vi "read_and_write.vi"() -> ()   [LabVIEW 2017]
uses:
  <vilib>/Platform/TimedLoop/XDataNode/timing_clust.ctl
  <vilib>/Platform/TimedLoop/XDataNode/nitl_modes.ctl
  <vilib>/Platform/TimedLoop/XDataNode/wakeup.ctl
  <vilib>/rvi/Emulation/niFpgaSctlEmulationGetInTimedLoop.vi
  <vilib>/rvi/Emulation/niFpgaProcessEmulError.vi
  <vilib>/rvi/Emulation/niFpgaGetClockAttributes.vi
  <vilib>/rvi/Emulation/niFpgaEmulationReportErrorSimple.vi
  <vilib>/rvi/eio/common/nirviEmuTemplateMethod_errors.vi
  <vilib>/rvi/interface/RandomDataEmulation/niFpgaRandomDataHandleErrors.vi
  <vilib>/rvi/Emulation/niFpgaCriticalErrorInLSC.vi
  <vilib>/eio/EIONode/EIONode.xnode
  <vilib>/rvi/DataTransferAndStorage/Container/XNode/niFpgaContainer.xnode
  <vilib>/rvi/interface/RandomDataEmulation/nirviRandomDataFpgaReadWriteTemplate.vi
  <vilib>/Platform/TimedLoop/XDataNode/XDataNode.xnode
  <vilib>/Platform/TimedLoop/XDataNode/XDNodeRunTimeDep.lvlib
panel:
  in  "stop":bool
  in  "safety catch":bool=TRUE
  in  "Timeout scope":i32
  out "timed out scope":bool=TRUE
  in  "power threshold (scope)":i32=80
  out "trigger":i16
  in  "count ticks scope":u32=8500
  in  "count ticks generating":u32=50000
  in  "Timeout err_check":i32
  in  "Timeout gen":i32
  out "timed out error_check":bool
  in  "count ticks reading":u32=500
  in  "minus x channel (gen)":i16
  in  "minus y channel (gen)":i16
  out "timed out gen":bool=TRUE
  in  "power (gen)":i16
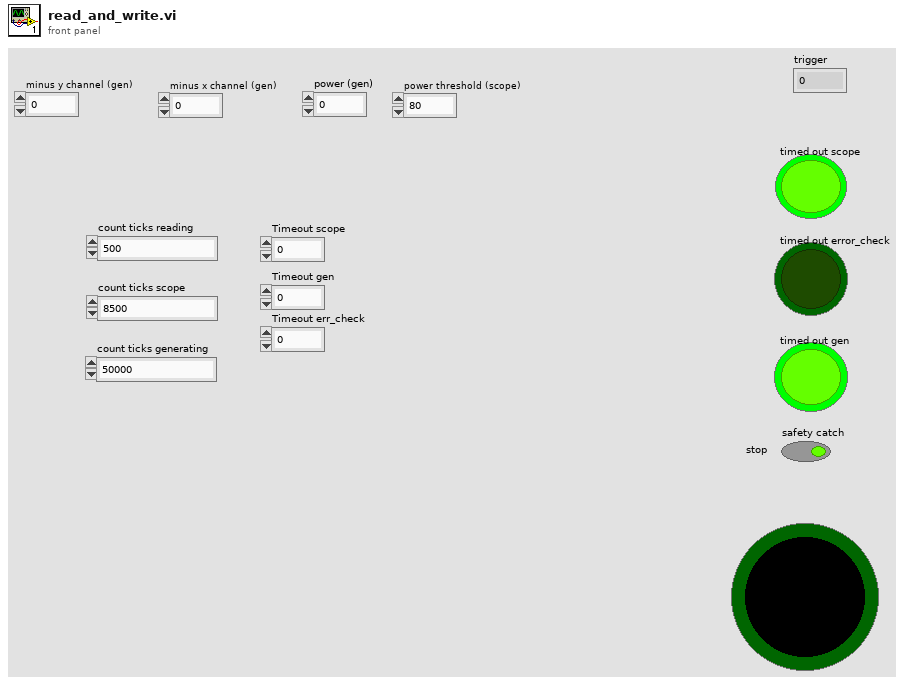
[diagram p1: front panel]
types:
  T1 = typedef "XDNodeRunTimeDep.lvlib/timing_clust.ctl" = cluster{"Expected End [f-1]":u64, "Actual End [f-1]":u64, "Finished Late? [f-1]":bool, "Expected End [i-1]":u64, "Actual End [i-1]":u64, "Finished Late? [i-1]":bool, "Expected Start [i]":u64, "Actual Start [i]":u64, "Expected Start [f]":u64, "Actual Start [f]":u64, "Source Name":string, "Structure Name":string, "Period":i64, "Deadline":i64, "Offset":i64, "Start":i64, "Priority":i32, "Timeout":i32, "Mode":T2, "Wakeup Reason":T3, "Error":errorcluster, "Source Type":string, "Secondary Source Type":string, "Global End Time":u64, "Global Start Time":u64, "Frame Duration":u64, "Iteration Duration":u64, "Assigned CPU":i32, "I/O Scan Engine Mode":u32}
  T2 = typedef "XDNodeRunTimeDep.lvlib/nitl_modes.ctl" = enum32{"No Change", "Process missed periods, maintain original phase", "Discard missed periods, maintain original phase", "Process missed periods, ignore original phase", "Discard missed periods, ignore original phase"}
  T3 = typedef "XDNodeRunTimeDep.lvlib/wakeup.ctl" = enum32{"Normal", "Aborted", "Asynchronous wakeup", "Timing source error", "Timed loop error", "Timeout"}
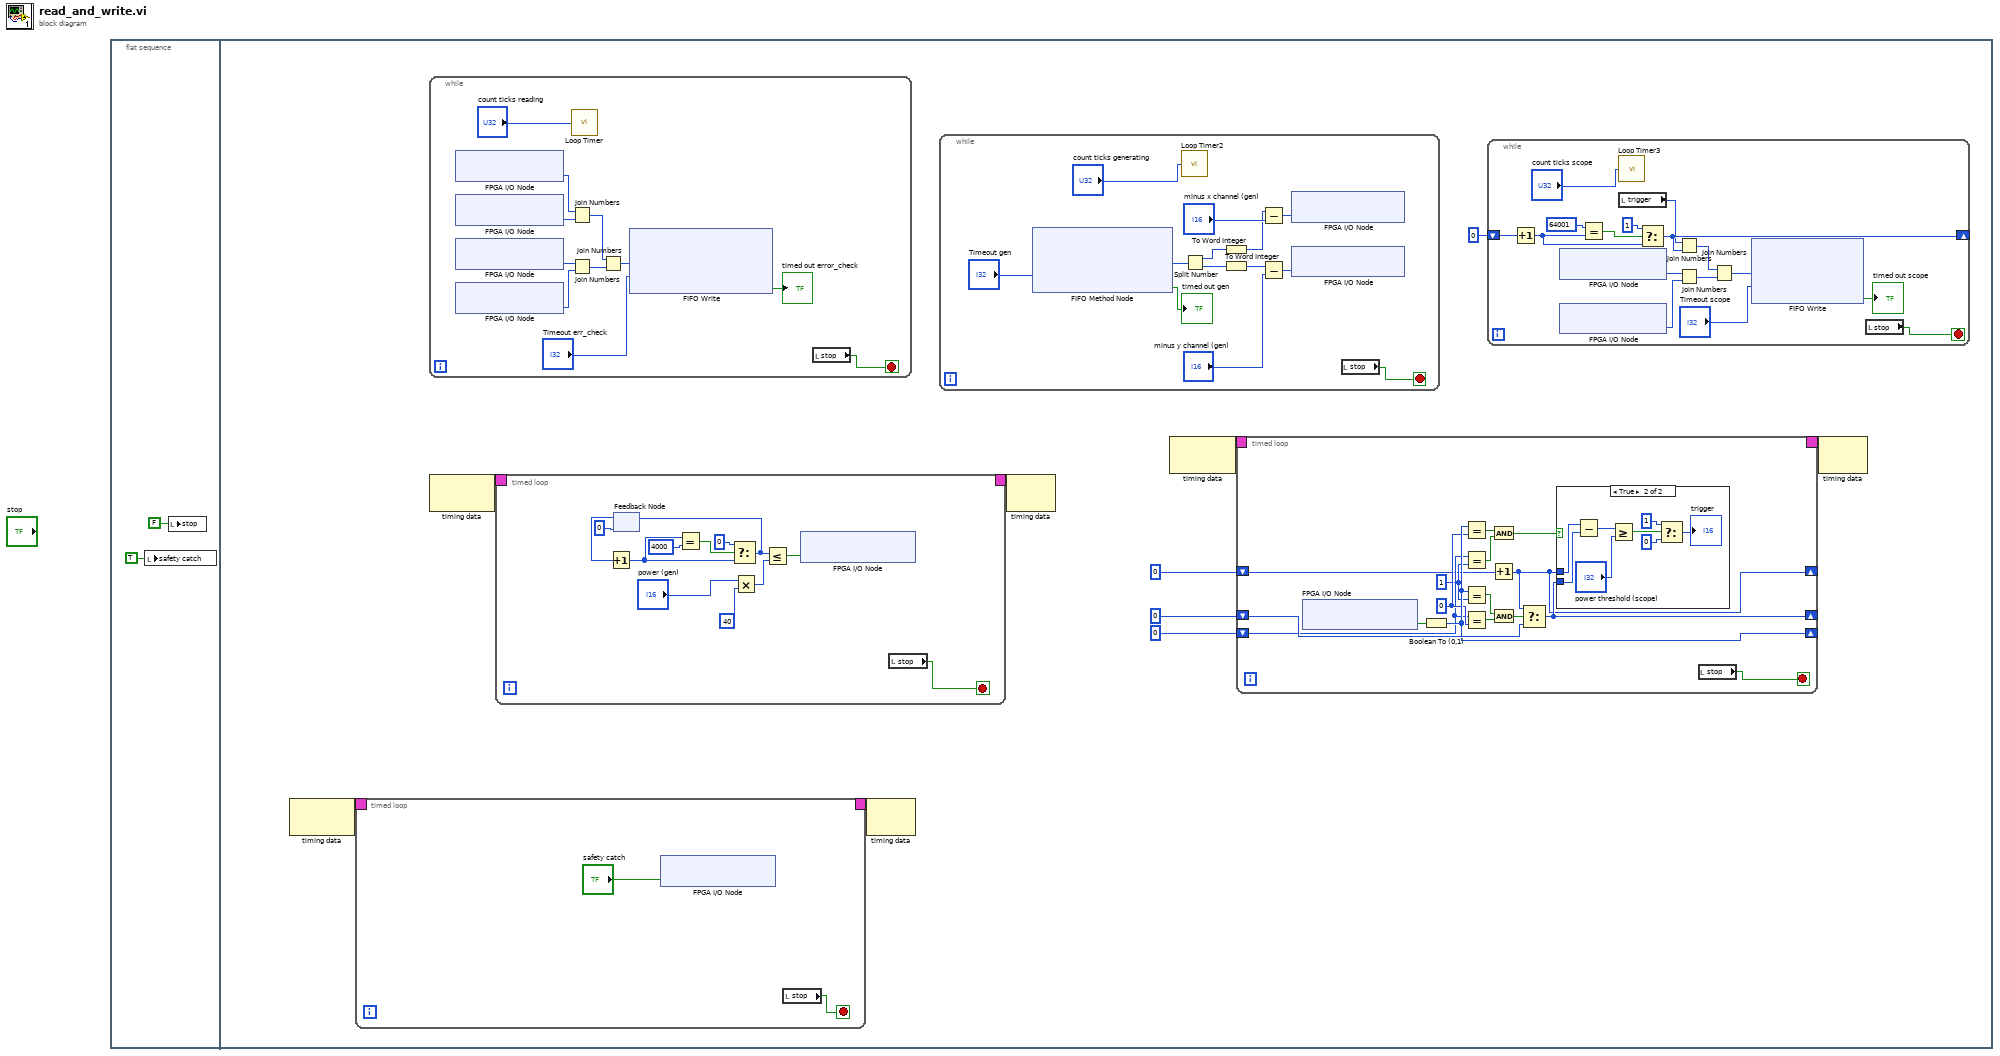
[diagram p0: block diagram]
diagram:
  n1 = flat-sequence {
    frame #0 {
      n2 = local write "safety catch"(TRUE ("safety catch")) -> ()
      n3 = local write "stop"(FALSE ("stop")) -> ()
    }
    frame #1 {
      n4 = node-c288() -> (w8:T1)  [unwired: 1 in]
      n5 = timed-loop {
        timing: w8 -> [_]
        timing-out: [_] -> w7
        stop <- w13 stop-if-true
        n6 = xnode "FPGA I/O Node"("ConnectorA/DIO2"="safety catch") -> ()  [unwired: 1 in, 1 out]
        n7 = local read "stop"() -> (w13:bool)
      }
      n8 = while {
        stop <- w92 stop-if-true
        n9 = xnode "FPGA I/O Node"() -> ("ConnectorA/AI0"=w101:u16)  [unwired: 1 in, 1 out]
        n10 = xnode "FPGA I/O Node"() -> ("ConnectorA/AI1"=w100:u16)  [unwired: 1 in, 1 out]
        n11 = xnode "FPGA I/O Node"() -> ("ConnectorA/AI2"=w99:u16)  [unwired: 1 in, 1 out]
        n12 = xnode "FPGA I/O Node"() -> ("ConnectorA/AI3"=w98:u16)  [unwired: 1 in, 1 out]
        n13 = Join Numbers(hi=w101, lo=w100) -> ((hi.lo)=w97:u32)
        n14 = Join Numbers(hi=w99, lo=w98) -> ((hi.lo)=w96:u32)
        n15 = call "Loop Timer"("Count(Ticks)"="count ticks reading") -> ()  [unwired: 1 out]
        n16 = Join Numbers(hi=w97, lo=w96) -> ((hi.lo)=w95:u64)
        n17 = xnode ("FIFO Write")("Element"=w95, "Timeout"="Timeout err_check") -> ("Timed Out?"=→"timed out error_check":bool)  [unwired: 1 in, 1 out]
        n18 = local read "stop"() -> (w92:bool)
      }
      n19 = node-c288() -> (w12:T1)  [unwired: 1 in]
      n20 = timed-loop {
        timing: w12 -> [_]
        timing-out: [_] -> w11
        stop <- w76 stop-if-true
        n21 = feedback #1(i16 0) -> (w87:i16)
        n22 = Increment(x=w87) -> (x+1=w79:i16)
        n23 = Equal?(x=w79, y=i16 4000) -> (x = y?=w82:bool)
        n24 = Select(t=i16 0, s=w82, f=w79) -> (s? t:f=w78:i16)
        n25 = feedback-in #1(w78) -> ()
        n26 = Multiply(x="power (gen)", y=i16 40) -> (x*y=w84:i16)
        n27 = Less Or Equal?(x=w78, y=w84) -> (x <= y?=w77:bool)
        n28 = xnode "FPGA I/O Node"("ConnectorA/DIO0"=w77) -> ()  [unwired: 1 in, 1 out]
        n29 = local read "stop"() -> (w76:bool)
      }
      n30 = node-c288(w7) -> ()  [unwired: 1 out]
      n31 = while {
        stop <- w63 stop-if-true
        n32 = xnode ("FIFO Method Node")("Timeout"="Timeout gen") -> ("Element"=w65:i32, "Timed Out?"=→"timed out gen":bool)  [unwired: 1 in, 1 out]
        n33 = call "Loop Timer2"("Count(Ticks)"="count ticks generating") -> ()  [unwired: 1 out]
        n34 = Split Number(x=w65) -> (hi(x)=w66:u16, lo(x)=w67:u16)
        n35 = To Word Integer(number=w66) -> (16bit integer=w68:i16)
        n36 = To Word Integer(number=w67) -> (16bit integer=w70:i16)
        n37 = Subtract(x=w68, y="minus x channel (gen)") -> (x-y=w72:i16)
        n38 = Subtract(x=w70, y="minus y channel (gen)") -> (x-y=w73:i16)
        n39 = xnode "FPGA I/O Node"("ConnectorC/AO0"=w72) -> ()  [unwired: 1 in, 1 out]
        n40 = xnode "FPGA I/O Node"("ConnectorC/AO1"=w73) -> ()  [unwired: 1 in, 1 out]
        n41 = local read "stop"() -> (w63:bool)
      }
      n42 = node-c288(w11) -> ()  [unwired: 1 out]
      n43 = node-c288() -> (w10:T1)  [unwired: 1 in]
      n44 = timed-loop {
        timing: w10 -> [_]
        timing-out: [_] -> w9
        shift-right: [w29] -> _
        shift-left: i16 0 -> [w27]
        shift-right: [w22] -> _
        shift-left: i16 0 -> [w30]
        shift-right: [w20] -> _
        shift-left: u64 0 -> [w21]
        stop <- w19 stop-if-true
        w28 = i16 0 ("y")
        w26 = i16 1 ("y")
        n45 = xnode "FPGA I/O Node"() -> ("ConnectorA/DIO4"=w34:bool)  [unwired: 1 in, 1 out]
        n46 = Boolean To (0,1)(Boolean=w34) -> (0, 1=w29:i16)
        n47 = Equal?(x=w29, y=w28) -> (x = y?=w24:bool)
        n48 = Equal?(x=w27, y=w26) -> (x = y?=w25:bool)
        n49 = Equal?(x=w29, y=w26) -> (x = y?=w33:bool)
        n50 = Equal?(x=w27, y=w28) -> (x = y?=w32:bool)
        n51 = Increment(x=w21) -> (x+1=w20:u64)
        n52 = And(x=w24, y=w25) -> (x .and. y?=w23:bool)
        n53 = And(x=w33, y=w32) -> (x .and. y?=w31:bool)
        n54 = Select(t=w20, s=w31, f=w30) -> (s? t:f=w22:u64)
        n55 = case shown="True" w23 {
          tunnel: w20 -> [_ w42]
          tunnel: w22 -> [_ w41]
          frame False {
          }
          frame True {
            n56 = Subtract(x=w42, y=w41) -> (x-y=w40:u64)
            n57 = Greater Or Equal?(x=w40, y="power threshold (scope)") -> (x >= y?=w38:bool)
            n58 = Select(t=i16 1, s=w38, f=i16 0) -> (s? t:f=→"trigger":i16)
          }
        }
        n59 = local read "stop"() -> (w19:bool)
      }
      n60 = while {
        shift-right: [w53] -> _
        shift-left: u16 0 -> [w58]
        stop <- w47 stop-if-true
        n61 = Increment(x=w58) -> (x+1=w54:u16)
        n62 = xnode "FPGA I/O Node"() -> ("ConnectorC/AI0"=w51:i16)  [unwired: 1 in, 1 out]
        n63 = xnode "FPGA I/O Node"() -> ("ConnectorC/AI1"=w52:i16)  [unwired: 1 in, 1 out]
        n64 = Equal?(x=u16 64001, y=w54) -> (x = y?=w56:bool)
        n65 = call "Loop Timer3"("Count(Ticks)"="count ticks scope") -> ()  [unwired: 1 out]
        n66 = local read "trigger"() -> (w50:i16)
        n67 = Select(t=u16 1, s=w56, f=w54) -> (s? t:f=w53:u16)
        n68 = Join Numbers(hi=w50, lo=w53) -> ((hi.lo)=w59:u32)
        n69 = Join Numbers(hi=w51, lo=w52) -> ((hi.lo)=w60:u32)
        n70 = Join Numbers(hi=w59, lo=w60) -> ((hi.lo)=w61:u64)
        n71 = xnode ("FIFO Write")("Element"=w61, "Timeout"="Timeout scope") -> ("Timed Out?"=→"timed out scope":bool)  [unwired: 1 in, 1 out]
        n72 = local read "stop"() -> (w47:bool)
      }
      n73 = node-c288(w9) -> ()  [unwired: 1 out]
    }
  }
